vi "ADO Connection Open by string.vi"(6 "Password":string, 7 "UserID":string, 8 "error in (no error)":errorcluster caption="错误输入（无错误）", 9 "connection timeout (15)":i32=15, 10 "ConnectionString":string, 11 "Database Connection 输入":refnum<class "Database Connection.lvclass"> caption="DNL_LabVIEW Object in") -> (0 "error out":errorcluster caption="错误输出", 3 "Database Connection 输出":refnum<class "Database Connection.lvclass"> caption="DNL_LabVIEW Object out")   [LabVIEW 2011, in "Database Connection.lvclass"]
uses:
  Database Connection.lvclass
  Database Connection.lvclass/Database Connection.ctl
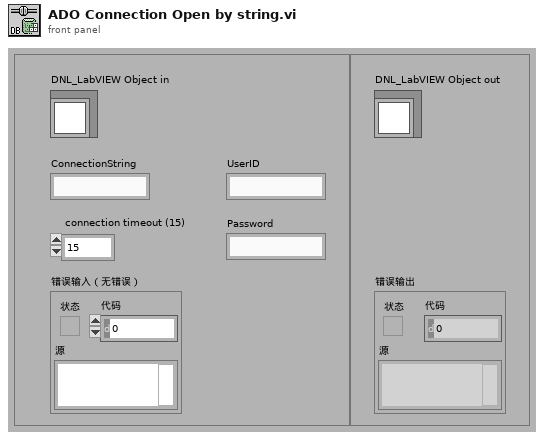
[diagram p1: front panel]
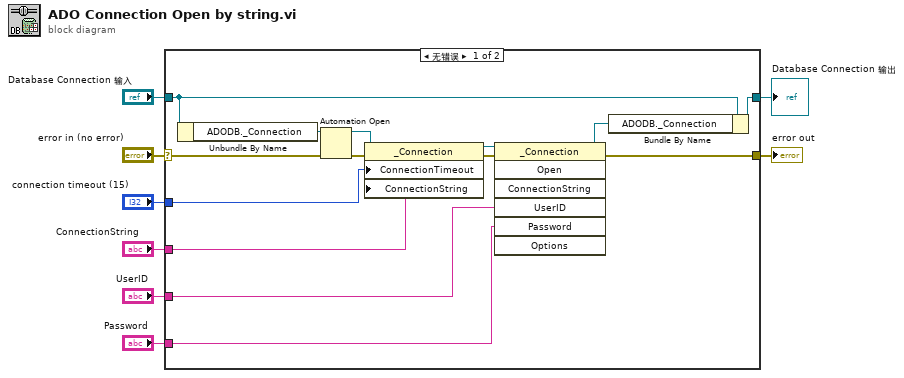
[diagram p0: block diagram]
diagram:
  n1 = case shown="无错误" "error in (no error)" {
    selector: "error in (no error)" -> [w22 w24]
    tunnel: [w10 w24] -> w7
    tunnel: [w13 w23] -> w5
    tunnel: "Database Connection 输入" -> [w12 w23]
    tunnel: "connection timeout (15)" -> [w16 _]
    tunnel: "ConnectionString" -> [w9 _]
    tunnel: "UserID" -> [w15 _]
    tunnel: "Password" -> [w14 _]
    frame No Error {
      n2 = Unbundle By Name(w12) -> ("ADODB._Connection"=w21:refnum<k7>)
      n3 = Automation Open(error in (no error)=w22, Automation Refnum=w21) -> (Automation Refnum=w20:refnum<k7>, error out=w18:errorcluster)  [unwired: 2 in]
      n4 = property class="_Connection"(reference=w20, error in=w18, "ConnectionTimeout"=w16, "ConnectionString"=w9) -> (reference out=w19:refnum<k7>, error out=w17:errorcluster)
      n5 = invoke class="_Connection" method="Open"(reference=w19, error in=w17, "UserID"=w15, "Password"=w14) -> (reference out=w11:refnum<k7>, error out=w10:errorcluster)  [unwired: 3 in, 5 out]
      n6 = Bundle By Name(cluster=w12, "ADODB._Connection"=w11) -> (w13:refnum<class "Database Connection.lvclass">)
    }
    frame Error {
    }
  }
  "error out" <- w7
  "Database Connection 输出" <- w5
